vi "lithographyMain.vi"() -> ()   [LabVIEW 2016]
uses:
  Controls/lithography_Control.ctl
  litho folder/Global/Lithography Data.vi
panel:
  out "Status":string
  out "Current Object":string
  in  "References":T1
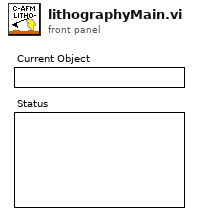
[diagram p1: front panel]
types:
  T1 = cluster{"Scan":refnum<k7>, "Litho":refnum<k7>, "Application":refnum<k7>}
  T2 = cluster{"X_offset":dbl, "Y_offset":dbl, "init_x":dbl, "init_y":dbl, "voltage":dbl}
  T3 = cluster{"Name":string, "Litho":cluster{"X":dbl, "Y":dbl, "Speed":dbl, "Voltage":dbl}[]}[]
  T4 = typedef "lithography_Control.ctl" = enum16{"open_app", "create_ref", "current_pos", "init_litho", "get_init_pt", "clear_litho", "set_param", "move_tip", "create_queue", "clean_up_litho", "start_litho", "end"}
  T5 = cluster{"References":cluster{"Scan":refnum<k7>, "Litho":refnum<k7>, "Application":refnum<k7>}, "Pattern Data":cluster{"Name":string, "Litho":cluster{"X":dbl, "Y":dbl, "Speed":dbl, "Voltage":dbl}[]}, "Values":cluster{"X_offset":dbl, "Y_offset":dbl, "init_x":dbl, "init_y":dbl, "voltage":dbl}}
  T6 = cluster{"X":dbl, "Y":dbl, "Speed":dbl, "Voltage":dbl}[]
  T7 = cluster{"X":dbl, "Y":dbl, "Speed":dbl, "Voltage":dbl}
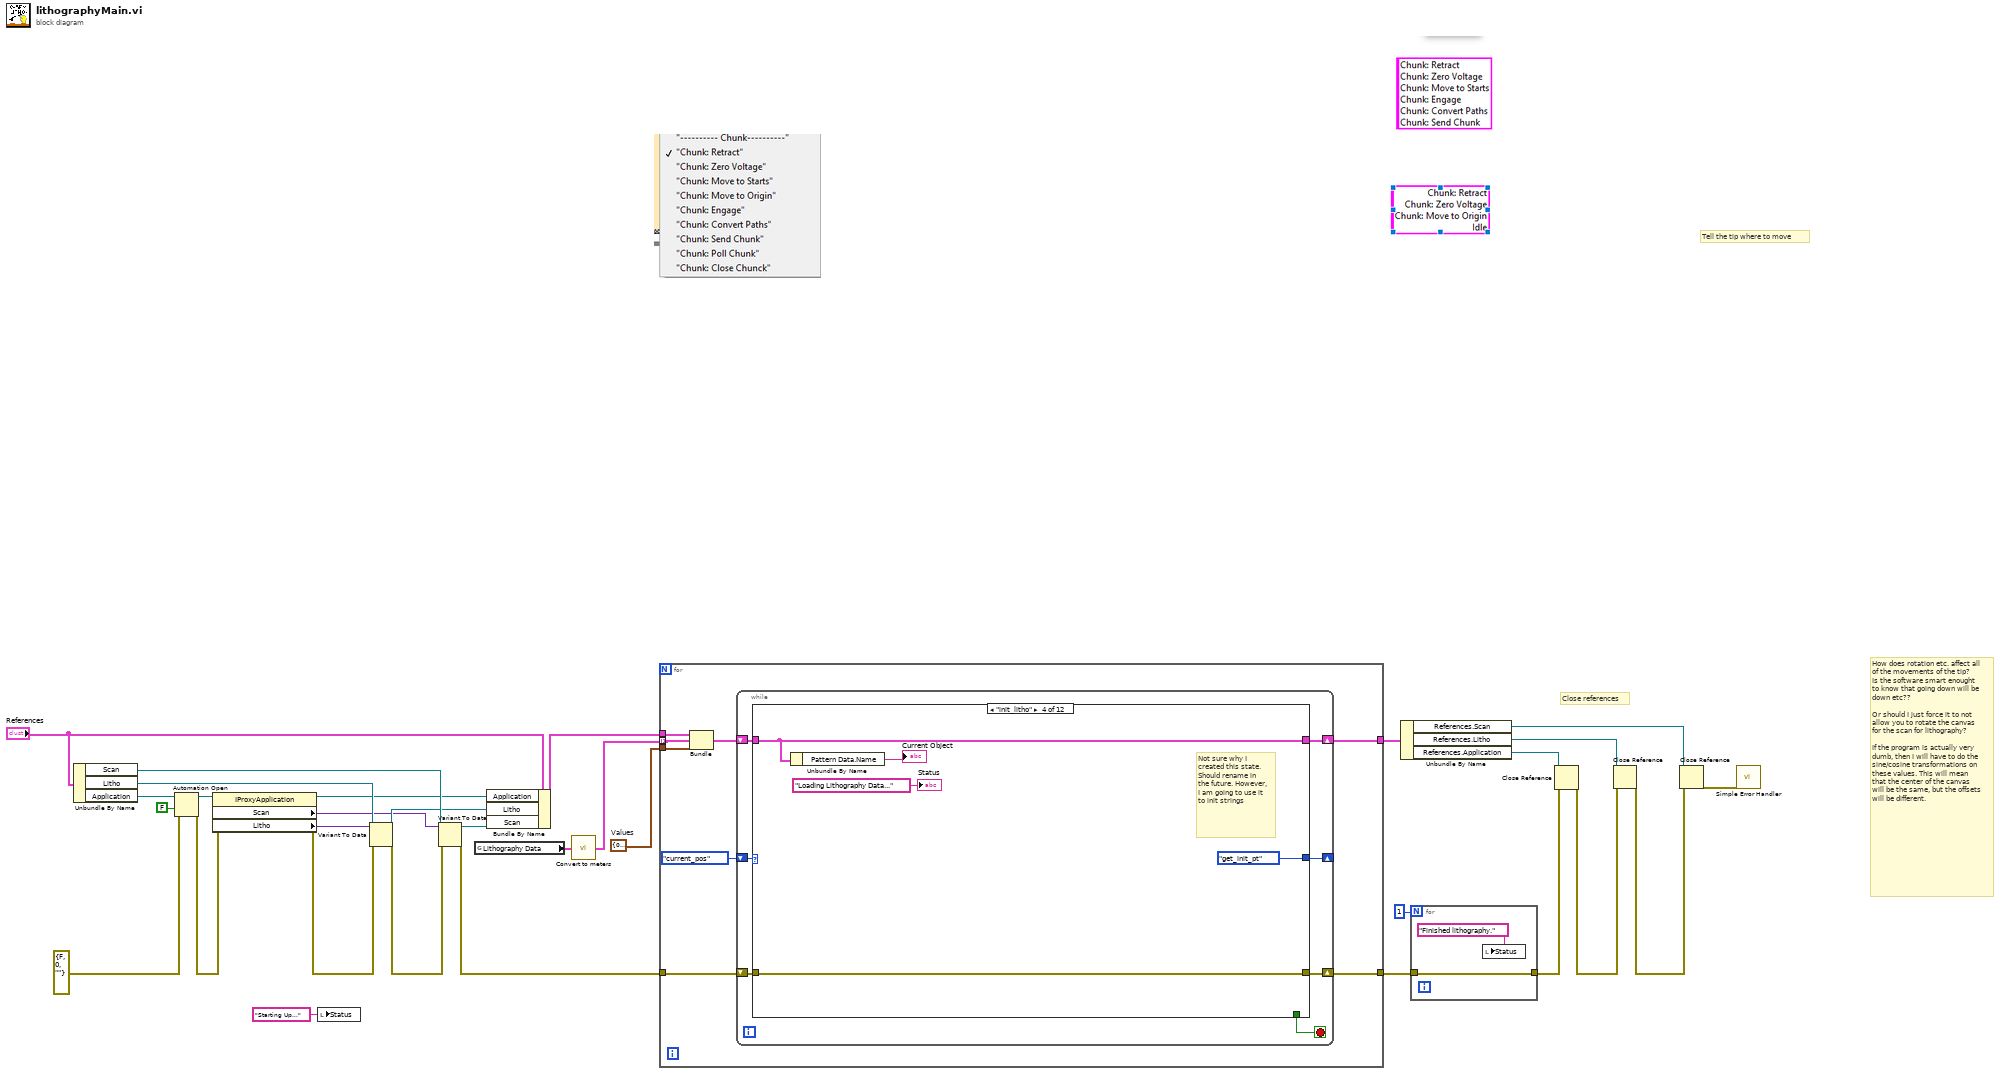
[diagram p0: block diagram]
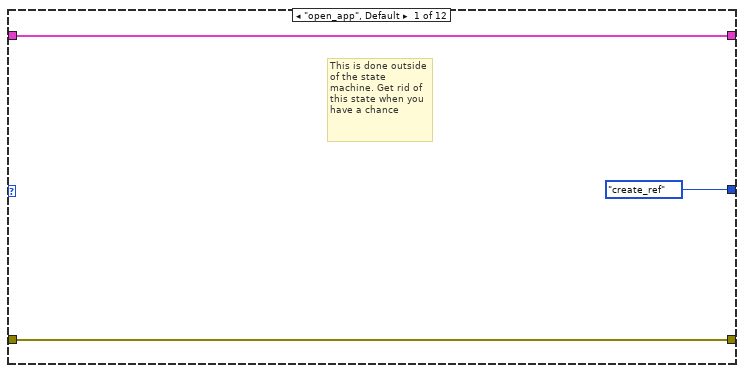
[diagram p2: hidden frame]
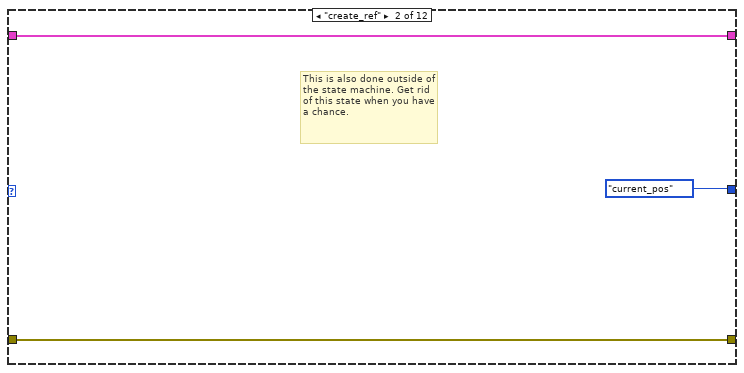
[diagram p3: hidden frame]
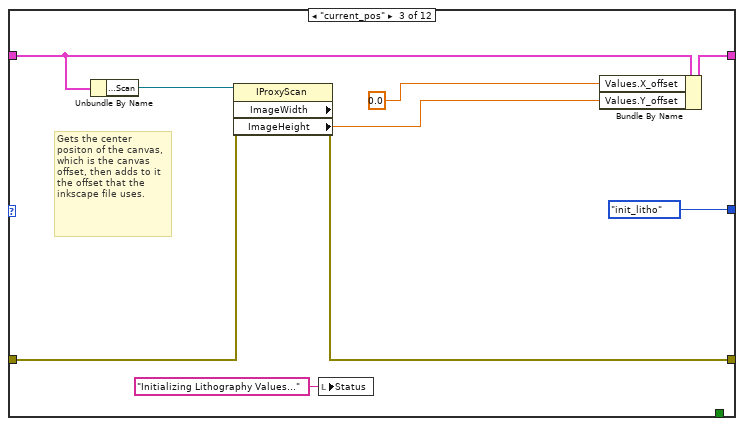
[diagram p4: hidden frame]
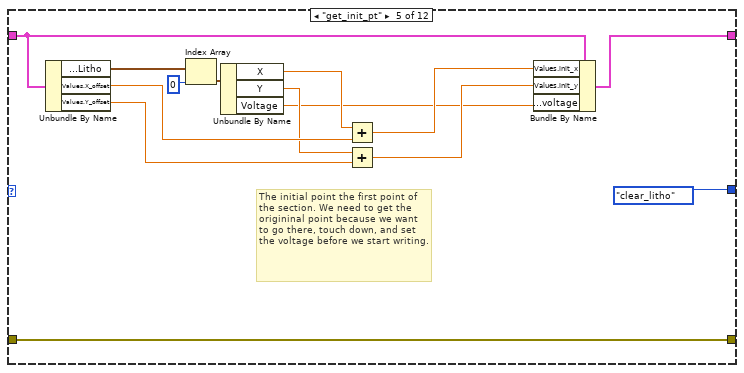
[diagram p5: hidden frame]
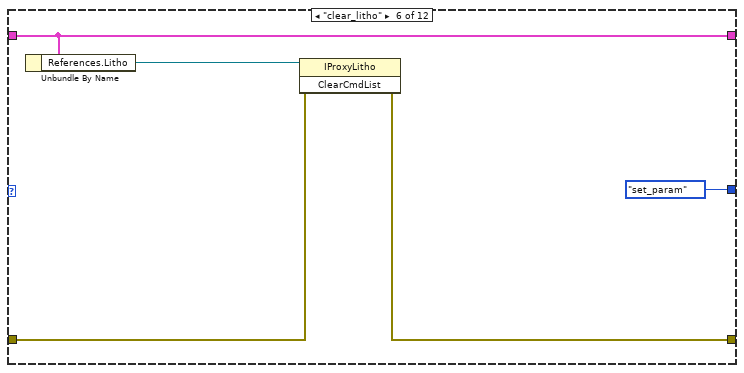
[diagram p6: hidden frame]
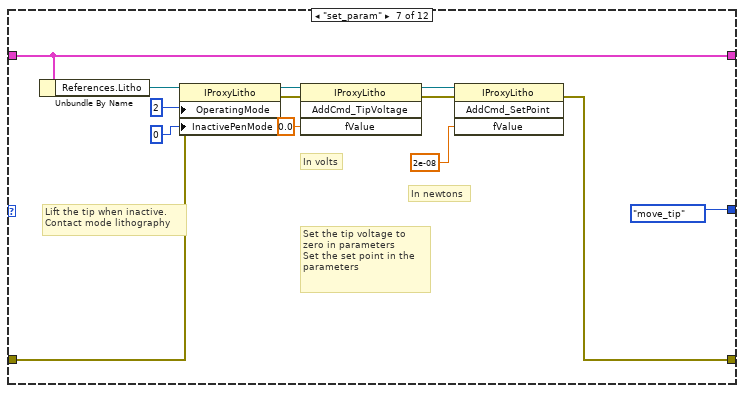
[diagram p7: hidden frame]
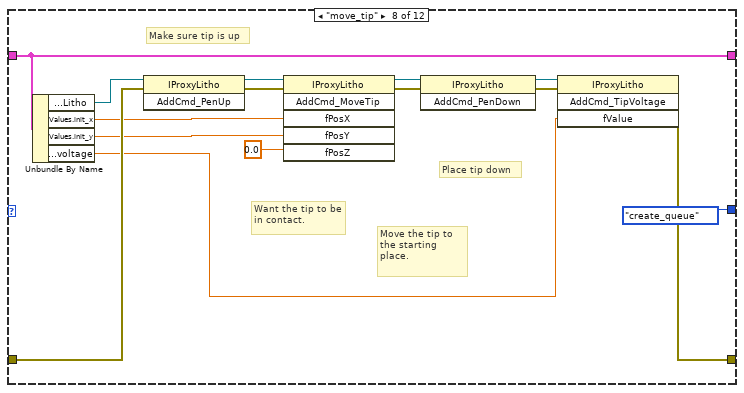
[diagram p8: hidden frame]
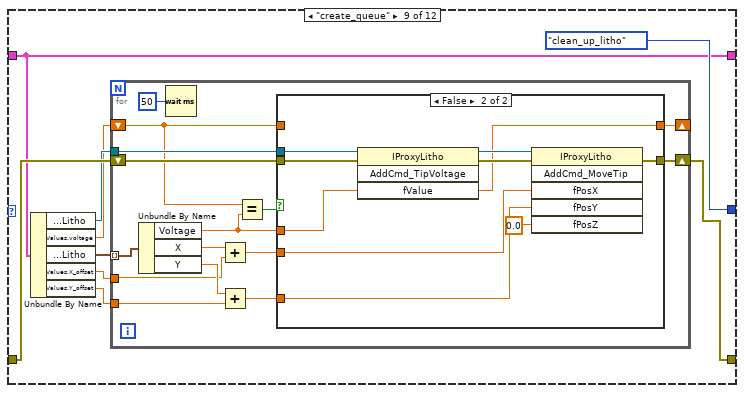
[diagram p9: hidden frame]
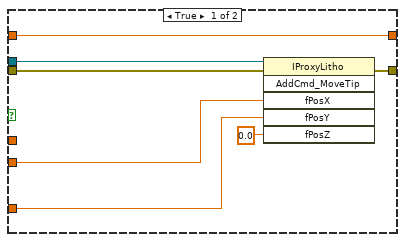
[diagram p10: hidden frame]
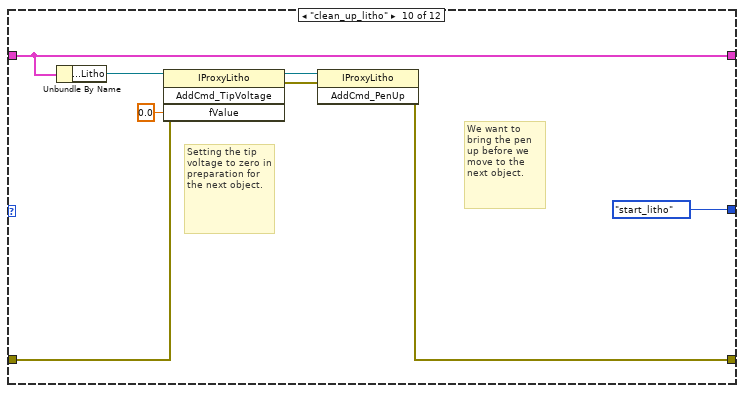
[diagram p11: hidden frame]
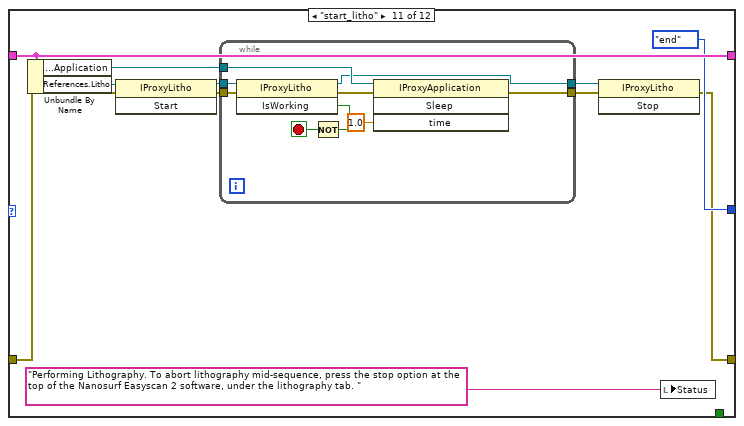
[diagram p12: hidden frame]
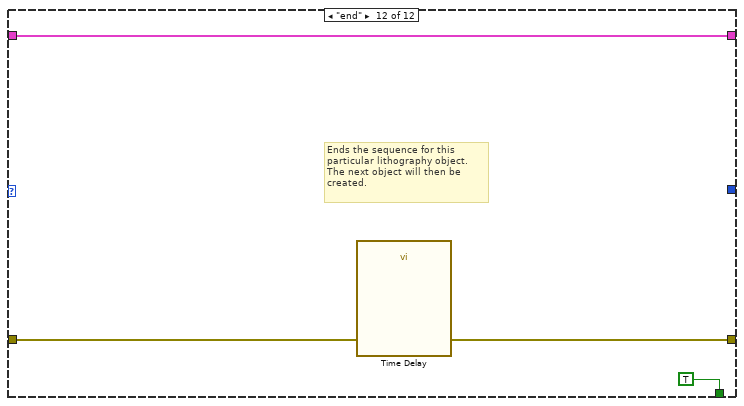
[diagram p13: hidden frame]
diagram:
  w31 = T2 {"X_offset"=0.0, "Y_offset"=0.0, "init_x"=0.0, "init_y"=0.0, "voltage"=0.0}  # Values
  # "Close references"
  # "How does rotation etc. affect all of the movements of the tip?\nIs the software smart enought to know that going down will be down etc??\n\nOr should I just force it to not allow you to rotate the canvas for the scan for lithography?\n\nIf the program is actually very dumb, then I will have to do the sine/cosine transformations on these values. This will mean that the center of the canvas will be the same, but the offsets will be different."
  # "Tell the tip where to move"
  n1 = Unbundle By Name("References") -> ("Scan"=w27:refnum<k7>, "Litho"=w28:refnum<k7>, "Application"=w29:refnum<k7>)
  n2 = Automation Open(error in (no error)=errorcluster {"status"=FALSE, "code"=0, "source"=""}, Automation Refnum=w29, 9:FALSE ("open new instance (false)")) -> (Automation Refnum=w30:refnum<k7>, error out=w13:errorcluster)  [unwired: 1 in]
  n3 = property class="IProxyApplication"(reference=w30, error in=w13) -> (reference out=w26:refnum<k7>, error out=w12:errorcluster, "Scan"=w17:variant, "Litho"=w16:variant)
  n4 = local write "Status"("Starting Up..." ("Status")) -> ()
  n5 = Variant To Data(error in=w12, type=w28, Variant=w16) -> (data=w25:refnum<k7>, error out=w11:errorcluster)
  n6 = Variant To Data(error in=w11, type=w27, Variant=w17) -> (data=w24:refnum<k7>, error out=w10:errorcluster)
  n7 = global read "Lithography Data.vi" "Lithography Data"() -> (w6:T3)
  n8 = Bundle By Name(cluster="References", "Application"=w26, "Litho"=w25, "Scan"=w24) -> (w23:T1)
  n9 = call "Convert to meters.vi"("Lithography Data In"=w6) -> ("Lithography Data Out"=w1:T3)
  n10 = for {
    tunnel: w23 -> [w37]
    tunnel: w1 -> [w38] mode=indexing
    tunnel: w10 -> [w36]
    tunnel: [w35] -> w3
    tunnel: w31 -> [w34]
    tunnel: [w33] -> w18
    n11 = Bundle("References"=w37, "Pattern Data"=w38, "Values"=w34) -> (w32:T5)  [unwired: 1 in]
    n12 = while {
      shift-right: [w42] -> _
      shift-left: lithography_Control."current_pos" -> [w46]
      shift-right: [w44] -> w33
      shift-left: w32 -> [w45]
      shift-right: [w41] -> w35
      shift-left: w36 -> [w43]
      stop <- w40 stop-if-true
      n13 = case shown="\"init_litho\"" w46 {
        tunnel: w45 -> [w47 w52 w59 w64 w71 w84 w97 w112 w119 w161 w173 w186]
        tunnel: [w47 w52 w58 w64 w70 w84 w97 w112 w119 w161 w173 w186] -> w44
        tunnel: w43 -> [w48 w50 w57 w65 w79 w82 w93 w106 w121 w156 w165 w183]
        tunnel: [lithography_Control."create_ref" lithography_Control."current_pos" lithography_Control."init_litho" lithography_Control."get_init_pt" lithography_Control."clear_litho" lithography_Control."set_param" lithography_Control."move_tip" lithography_Control."create_queue" lithography_Control."clean_up_litho" lithography_Control."start_litho" lithography_Control."end" _] -> w42
        tunnel: [w48 w50 w56 w65 w79 w81 w87 w101 w120 w160 w164 w184] -> w41
        tunnel: [_ _ _ _ _ _ _ _ _ _ _ TRUE] -> w40
        frame "open_app", Default {
          # "This is done outside of the state machine. Get rid of this state when you have a chance"
        }
        frame "create_ref" {
          # "This is also done outside of the state machine. Get rid of this state when you have a chance."
        }
        frame "current_pos" {
          # "Gets the center positon of the canvas, which is the canvas offset, then adds to it the offset that the inkscape file uses."
          n14 = Unbundle By Name(w59) -> ("References.Scan"=w60:refnum<k7>)
          n15 = property class="IProxyScan" props=["ImageWidth", "ImageHeight"](reference=w60, error in=w57) -> (error out=w56:errorcluster, "ImageHeight"=w54:dbl)  [unwired: 2 out]
          n16 = local write "Status"("Initializing Lithography Values..." ("Status")) -> ()
          n17 = Bundle By Name(cluster=w59, "Values.X_offset"=0.0 ("ImageWidth"), "Values.Y_offset"=w54) -> (w58:T5)
        }
        frame "init_litho" {
          # "Not sure why I created this state. Should rename in the future. However, I am going to use it to init strings"
          n18 = Unbundle By Name(w64) -> ("Pattern Data.Name"=→"Current Object":string)
          "Status" <- "Loading Lithography Data..." ("Status")
        }
        frame "get_init_pt" {
          # "The initial point the first point of the section. We need to get the origininal point because we want to go there, touch down, and set the voltage before we start writing."
          n19 = Unbundle By Name(w71) -> ("Pattern Data.Litho"=w77:T6, "Values.X_offset"=w74:dbl, "Values.Y_offset"=w72:dbl)
          n20 = Index Array(array=w77, index=0) -> (element=w76:T7)
          n21 = Unbundle By Name(w76) -> ("X"=w75:dbl, "Y"=w73:dbl, "Voltage"=w67:dbl)
          n22 = Add(x=w75, y=w74) -> (x+y=w69:dbl)
          n23 = Add(x=w73, y=w72) -> (x+y=w68:dbl)
          n24 = Bundle By Name(cluster=w71, "Values.init_x"=w69, "Values.init_y"=w68, "Values.voltage"=w67) -> (w70:T5)
        }
        frame "clear_litho" {
          n25 = Unbundle By Name(w84) -> ("References.Litho"=w83:refnum<k7>)
          n26 = invoke class="IProxyLitho" method="ClearCmdList"(reference=w83, error in=w82) -> (error out=w81:errorcluster)  [unwired: 1 in, 2 out]
        }
        frame "set_param" {
          # "In volts"
          # "In newtons"
          # "Set the tip voltage to zero in parameters\nSet the set point in the parameters"
          # "Lift the tip when inactive.\nContact mode lithography"
          n27 = Unbundle By Name(w97) -> ("References.Litho"=w96:refnum<k7>)
          n28 = property class="IProxyLitho"(reference=w96, error in=w93, "OperatingMode"=2 ("InactivePenMode"), "InactivePenMode"=0 ("OperatingMode")) -> (reference out=w92:refnum<k7>, error out=w91:errorcluster)
          n29 = invoke class="IProxyLitho" method="AddCmd_TipVoltage"(reference=w92, error in=w91, "fValue"=0.0) -> (reference out=w89:refnum<k7>, error out=w88:errorcluster)  [unwired: 1 in, 2 out]
          n30 = invoke class="IProxyLitho" method="AddCmd_SetPoint"(reference=w89, error in=w88, "fValue"=2e-08 ("SetPoint")) -> (error out=w87:errorcluster)  [unwired: 1 in, 3 out]
        }
        frame "move_tip" {
          # "Want the tip to be in contact."
          # "Make sure tip is up"
          # "Place tip down"
          # "Move the tip to the starting place."
          n31 = Unbundle By Name(w112) -> ("References.Litho"=w105:refnum<k7>, "Values.init_x"=w104:dbl, "Values.init_y"=w103:dbl, "Values.voltage"=w99:dbl)
          n32 = invoke class="IProxyLitho" method="AddCmd_PenUp"(reference=w105, error in=w106) -> (reference out=w111:refnum<k7>, error out=w108:errorcluster)  [unwired: 1 in, 1 out]
          n33 = invoke class="IProxyLitho" method="AddCmd_MoveTip"(reference=w111, error in=w108, "fPosX"=w104, "fPosY"=w103, "fPosZ"=0.0) -> (reference out=w110:refnum<k7>, error out=w107:errorcluster)  [unwired: 1 in, 4 out]
          n34 = invoke class="IProxyLitho" method="AddCmd_PenDown"(reference=w110, error in=w107) -> (reference out=w102:refnum<k7>, error out=w100:errorcluster)  [unwired: 1 in, 1 out]
          n35 = invoke class="IProxyLitho" method="AddCmd_TipVoltage"(reference=w102, error in=w100, "fValue"=w99) -> (error out=w101:errorcluster)  [unwired: 1 in, 3 out]
        }
        frame "create_queue" {
          n36 = Unbundle By Name(w119) -> ("References.Litho"=w115:refnum<k7>, "Values.voltage"=w114:dbl, "Pattern Data.Litho"=w118:T6, "Values.X_offset"=w117:dbl, "Values.Y_offset"=w116:dbl)
          n37 = for {
            shift-right: [w135] -> w120
            shift-left: w121 -> [w136]
            tunnel: w115 -> [w137]
            tunnel: w118 -> [w127] mode=indexing
            tunnel: w117 -> [w128]
            tunnel: w116 -> [w132]
            shift-right: [w124] -> _
            shift-left: w114 -> [w123]
            n38 = Unbundle By Name(w127) -> ("Voltage"=w125:dbl, "X"=w134:dbl, "Y"=w131:dbl)
            n39 = Wait (ms)(milliseconds to wait=u32 50) -> ()  [unwired: 1 out]
            n40 = Add(x=w134, y=w128) -> (x+y=w133:dbl)
            n41 = Add(x=w131, y=w132) -> (x+y=w130:dbl)
            n42 = Equal?(x=w123, y=w125) -> (x = y?=w126:bool)
            n43 = case shown="False" w126 {
              tunnel: w137 -> [w144 w150]
              tunnel: w136 -> [w143 w149]
              tunnel: [w141 w153] -> w135
              tunnel: w133 -> [w140 w152]
              tunnel: w130 -> [w139 w151]
              tunnel: w125 -> [_ w146]
              tunnel: [w138 w145] -> w124
              tunnel: w123 -> [w138 _]
              frame True {
                n44 = invoke class="IProxyLitho" method="AddCmd_MoveTip"(reference=w144, error in=w143, "fPosX"=w140, "fPosY"=w139, "fPosZ"=0.0 ("fPosX")) -> (error out=w141:errorcluster)  [unwired: 1 in, 5 out]
              }
              frame False {
                n45 = invoke class="IProxyLitho" method="AddCmd_TipVoltage"(reference=w150, error in=w149, "fValue"=w146) -> (reference out=w147:refnum<k7>, error out=w148:errorcluster, "fValue"=w145:dbl)  [unwired: 1 in, 1 out]
                n46 = invoke class="IProxyLitho" method="AddCmd_MoveTip"(reference=w147, error in=w148, "fPosX"=w152, "fPosY"=w151, "fPosZ"=0.0 ("fPosX")) -> (error out=w153:errorcluster)  [unwired: 1 in, 5 out]
              }
            }
          }
        }
        frame "clean_up_litho" {
          # "Setting the tip voltage to zero in preparation for the next object."
          # "We want to bring the pen up before we move to the next object."
          n47 = Unbundle By Name(w161) -> ("References.Litho"=w159:refnum<k7>)
          n48 = invoke class="IProxyLitho" method="AddCmd_TipVoltage"(reference=w159, error in=w156, "fValue"=0.0) -> (reference out=w158:refnum<k7>, error out=w157:errorcluster)  [unwired: 1 in, 2 out]
          n49 = invoke class="IProxyLitho" method="AddCmd_PenUp"(reference=w158, error in=w157) -> (error out=w160:errorcluster)  [unwired: 1 in, 2 out]
        }
        frame "start_litho" {
          n50 = Unbundle By Name(w173) -> ("References.Application"=w163:refnum<k7>, "References.Litho"=w172:refnum<k7>)
          n51 = invoke class="IProxyLitho" method="Start"(reference=w172, error in=w165) -> (reference out=w171:refnum<k7>, error out=w168:errorcluster)  [unwired: 1 in, 1 out]
          n52 = while {
            tunnel: w171 -> [w182]
            tunnel: [w174] -> w167
            tunnel: w168 -> [w180]
            tunnel: [w177] -> w166
            tunnel: w163 -> [w176]
            stop <- w179 stop-if-true
            n53 = invoke class="IProxyLitho" method="IsWorking"(reference=w182, error in=w180) -> (reference out=w174:refnum<k7>, error out=w178:errorcluster, "IsWorking"=w181:bool)  [unwired: 1 in]
            n54 = Not(x=w181) -> (.not. x?=w179:bool)
            n55 = invoke class="IProxyApplication" method="Sleep"(reference=w176, error in=w178, "time"=1.0) -> (error out=w177:errorcluster)  [unwired: 1 in, 3 out]
          }
          n56 = invoke class="IProxyLitho" method="Stop"(reference=w167, error in=w166) -> (error out=w164:errorcluster)  [unwired: 1 in, 2 out]
          n57 = local write "Status"("Performing Lithography. To abort lithography mid-sequence, press the stop option at the top of the Nanosurf Easyscan 2 software, under the lithography tab. " ("Status")) -> ()
        }
        frame "end" {
          # "Ends the sequence for this particular lithography object. The next object will then be created."
          n58 = call "Time Delay"("error in (no error)"=w183) -> ("error out"=w184:errorcluster)  [unwired: 10 in]
        }
      }
    }
  }
  n59 = Unbundle By Name(w18) -> ("References.Scan"=w19:refnum<k7>, "References.Litho"=w20:refnum<k7>, "References.Application"=w21:refnum<k7>)
  n60 = for {
    N: 1 -> [_]
    tunnel: w3 -> [w187]
    tunnel: [w187] -> w2
    n61 = local write "Status"("Finished lithography.") -> ()
  }
  n62 = Close Reference(reference=w21, error in (no error)=w2) -> (error out=w9:errorcluster)
  n63 = Close Reference(reference=w20, error in (no error)=w9) -> (error out=w8:errorcluster)
  n64 = Close Reference(reference=w19, error in (no error)=w8) -> (error out=w7:errorcluster)
  n65 = call <vilib>:"Simple Error Handler.vi"("error in (no error)"=w7) -> ()  [unwired: 4 in, 5 out]
